vi "Destroy image array.vi"(8 "error in (no error)":errorcluster, 11 "Image array":T1[](array[typedef])) -> (0 "error out":errorcluster)   [LabVIEW 2020]
doc: "Destroy all buffers contained in the input image array. If all images in the application need to be destroyed, use IMAQ Clear with All images? set to True."
uses:
  <vilib>/vision/Image Controls.llb/IMAQ Image.ctl
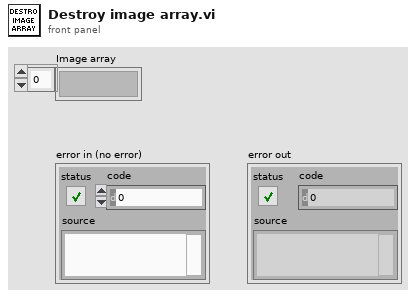
[diagram p1: front panel]
types:
  T1 = typedef "IMAQ Image.ctl" = refnum<image>
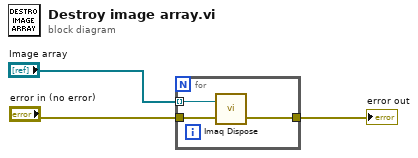
[diagram p0: block diagram]
diagram:
  n1 = for {
    tunnel: "Image array" -> [w6] mode=indexing
    tunnel: "error in (no error)" -> [w5]
    tunnel: [w4] -> w3
    n2 = call "Imaq Dispose"("Image"=w6, "error in (no error)"=w5) -> ("error out"=w4:errorcluster)  [unwired: 4 in]
  }
  "error out" <- w3
